vi "Hyperspectral Camera.vi"(7 "Photo Period (ms)":u32=2000, 8 "error in":errorcluster, 9 "Photo Save Directory":path, 10 "Hyperspectral Camera Session":T1, 11 "Notifier":refnum<notifier>) -> (0 "error out":errorcluster)   [LabVIEW 2025]
doc: "Main VI for handling hyperspectral camera."
uses:
  <vilib>/userDefined/High Color/IMAQdx.ctl
  defs/Notification Definition.ctl
  <vilib>/vision/driver/IMAQdx.llb/IMAQdx Acquisition Mode.ctl
  <vilib>/vision/driver/IMAQdx.llb/IMAQdx Buffer Number Mode.ctl
  <vilib>/vision/driver/NI_Vision_Acquisition_Software.lvlib
  <resource>/objmgr/imaqdx.rc
panel:
  out "DeviceModelName":string
  out "Last Taken Image":T2(plugin-control)
  in  "Stop":bool
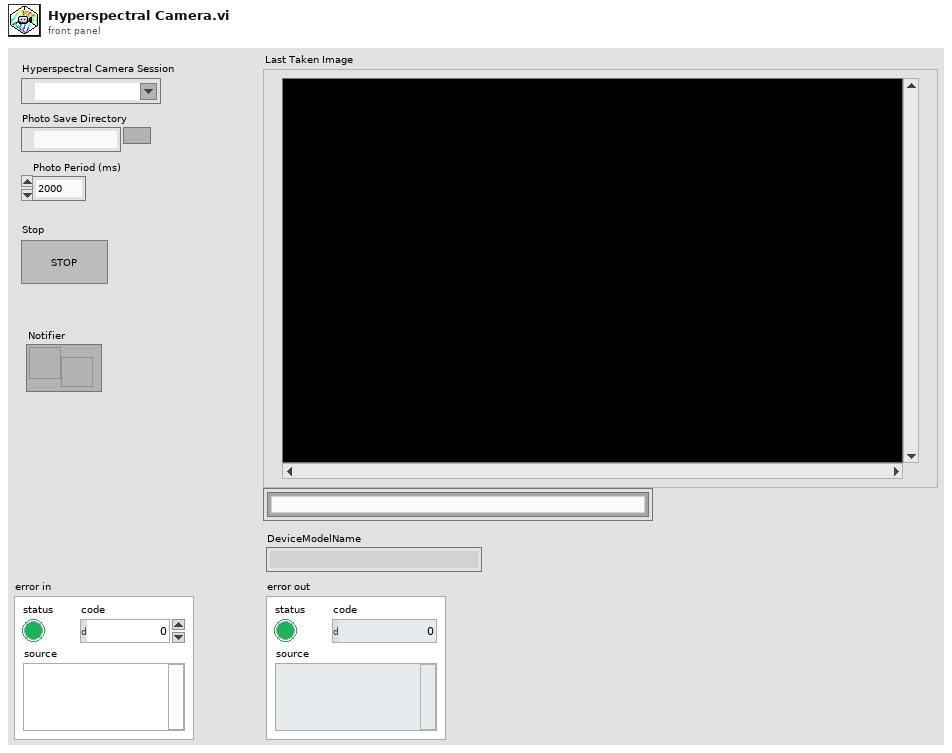
[diagram p1: front panel]
types:
  T1 = typedef "IMAQdx.ctl" = refnum<k21>
  T2 = typedef "IMAQ Image.ctl" = refnum<image>
  T3 = typedef "NI_Vision_Acquisition_Software.lvlib/IMAQdx Acquisition Mode.ctl" = enum32{"One Shot", "Continuous"}
  T4 = typedef "Image Type" = u32
  T5 = typedef "NI_Vision_Acquisition_Software.lvlib/IMAQdx Buffer Number Mode.ctl" = enum32{"Next", "Last", "Buffer Number", "Every", "Last New"}
  T6 = typedef "Notification Definition.ctl" = cluster{"Message":string}
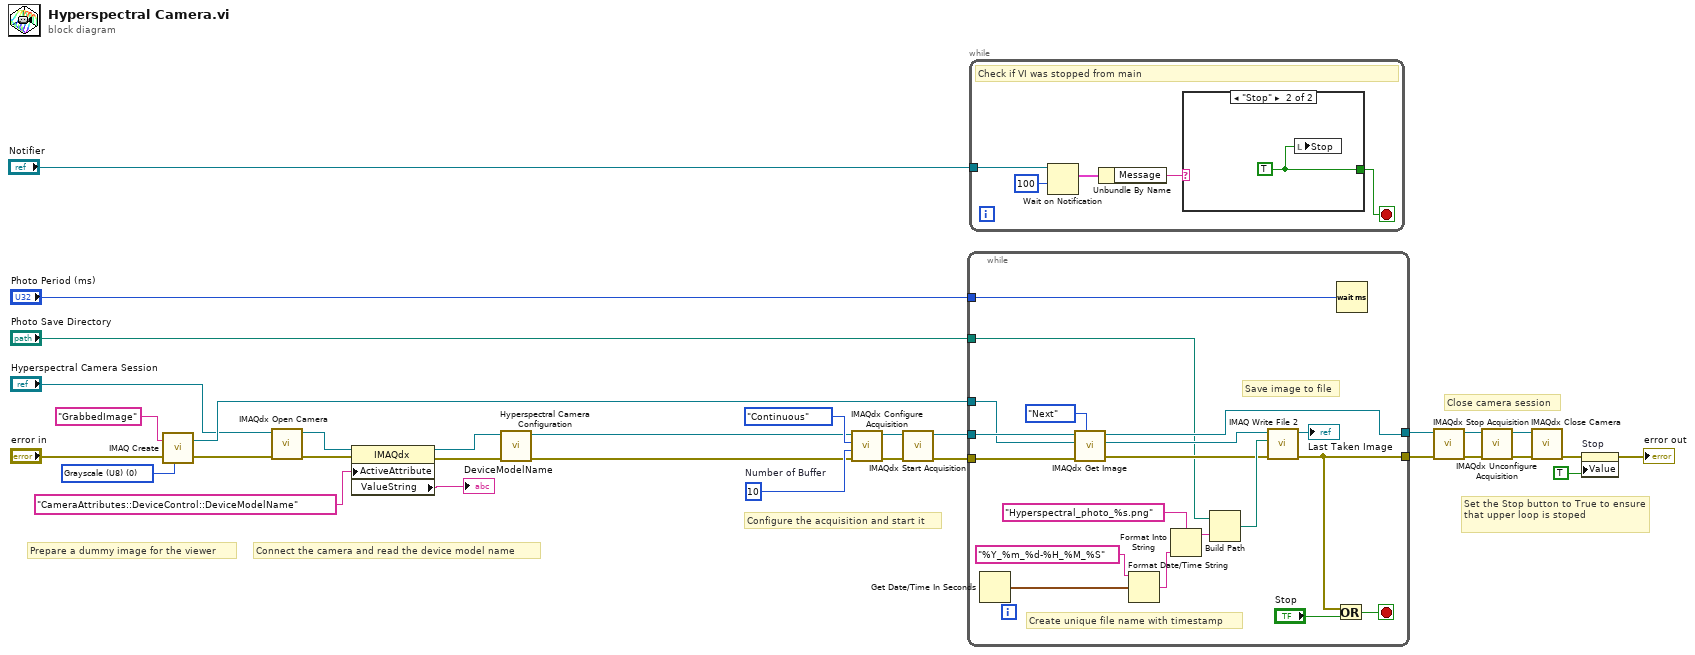
[diagram p0: block diagram]
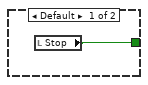
[diagram p2: hidden frame]
diagram:
  w14 = T4 0 items=["Grayscale (U8)", "Grayscale (I16)", "Grayscale (SGL)", "Complex (CSG)", "RGB (U32)", "HSL (U32)", "RGB (U64)", "Grayscale (U16)"] ("Image Type")
  w19 = u32 10  # Number of Buffer
  # "Set the Stop button to True to ensure that upper loop is stoped"
  # "Close camera session"
  # "Configure the acquisition and start it"
  # "Connect the camera and read the device model name"
  # "Prepare a dummy image for the viewer"
  n1 = call "IMAQ Create"("Image Name"="GrabbedImage", "Image Type"=w14, "error in (no error)"="error in") -> ("New Image"=w21:T2, "error out"=w22:errorcluster)  [unwired: 1 in, 1 out]
  n2 = call <vilib>:"IMAQdx Open Camera.vi"("error in"=w22, "Session In"="Hyperspectral Camera Session") -> ("error out"=w18:errorcluster, "Session Out"=w20:T1)  [unwired: 8 in]
  n3 = property on="Property Node" class="IMAQdx"(reference=w20, error in=w18, "ActiveAttribute"="CameraAttributes::DeviceControl::DeviceModelName") -> (reference out=w7:T1, error out=w5:errorcluster, "ValueString"=→"DeviceModelName":string)
  n4 = call "Hyperspectral Camera Configuration.vi"("error in"=w5, "Camera Session"=w7) -> ("error out"=w4:errorcluster, "Camera Session out"=w6:T1)  [unwired: 8 in]
  n5 = call <vilib>:"IMAQdx Configure Acquisition.vi"("error in"=w4, "Number of Buffers"=w19, "Continuous?"=IMAQdx_Acquisition_Mode."Continuous", "Session In"=w6) -> ("error out"=w32:errorcluster, "Session Out"=w31:T1)  [unwired: 6 out]
  n6 = call <vilib>:"IMAQdx Start Acquisition.vi"("error in"=w32, "Session In"=w31) -> ("error out"=w8:errorcluster, "Session Out"=w30:T1)  [unwired: 8 out]
  n7 = while {
    tunnel: w8 -> [w50]
    tunnel: w30 -> [w51]
    tunnel: w21 -> [w48]
    tunnel: [w41] -> w25
    tunnel: [w38] -> w24
    tunnel: "Photo Save Directory" -> [w37]
    tunnel: "Photo Period (ms)" -> [w36]
    stop <- w47 stop-if-true
    # "Create unique file name with timestamp"
    # "Save image to file"
    n8 = Get Date/Time In Seconds() -> (seconds since 1Jan1904=w35:timestamp)
    n9 = call <vilib>:"IMAQdx Get Image.vi"("Buffer Number Mode (Next)"=IMAQdx_Buffer_Number_Mode."Next", "error in"=w50, "Image In"=w48, "Session In"=w51) -> ("error out"=w43:errorcluster, "Image Out"=w45:T2, "Session Out"=w38:T1)  [unwired: 4 in, 1 out]
    n10 = Format Date/Time String(time format string (%c)="%Y_%m_%d-%H_%M_%S", seconds (now)=w35) -> (date/time string=w33:string)  [unwired: 1 in]
    n11 = Format Into String(format string="Hyperspectral_photo_%s.png", w33) -> (resulting string=w39:string)  [unwired: 2 in, 1 out]
    n12 = Build Path(base path=w37, name or relative path=w39) -> (appended path=w44:path)
    n13 = call-poly "IMAQ Write File 2"("error in (no error)"=w43, "File Path"=w44, "Image"=w45) -> ("error out"=w41:errorcluster, "Image Out (duplicate)"=→"Last Taken Image":T2)  [unwired: 7 in]
    n14 = Or(x=w41, y="Stop") -> (x .or. y?=w47:bool)
    n15 = Wait (ms)(milliseconds to wait=w36) -> ()  [unwired: 1 out]
  }
  n16 = while {
    tunnel: "Notifier" -> [w56]
    stop <- w53 stop-if-true
    # "Check if VI was stopped from main"
    n17 = Wait on Notification(notifier=w56, timeout in ms (-1)=100) -> (notification=w55:T6)  [unwired: 2 in, 3 out]
    n18 = Unbundle By Name(w55) -> ("Message"=w54:string)
    n19 = case shown="\"Stop\"" w54 {
      tunnel: [w57 w58] -> w53
      frame Default {
        n20 = local read "Stop"() -> (w57:bool)
      }
      frame "Stop" {
        w58 = TRUE
        n21 = local write "Stop"(w58) -> ()
      }
    }
  }
  n22 = call <vilib>:"IMAQdx Stop Acquisition.vi"("error in"=w25, "Session In"=w24) -> ("error out"=w29:errorcluster, "Session Out"=w28:T1)  [unwired: 8 out]
  n23 = call <vilib>:"IMAQdx Unconfigure Acquisition.vi"("error in"=w29, "Session In"=w28) -> ("error out"=w26:errorcluster, "Session Out"=w27:T1)  [unwired: 8 out]
  n24 = call <vilib>:"IMAQdx Close Camera.vi"("error in"=w26, "Session In"=w27) -> ("error out"=w3:errorcluster)  [unwired: 9 out]
  n25 = property on="Stop" class="Bool (strict)"(error in=w3, "Value"=TRUE ("Stop")) -> (error out=→"error out":errorcluster)  [unwired: 1 in, 1 out]
